vi "createPubDataEvents.vi"(8 "error in (no error)":errorcluster, 11 "PubSubDataEvent in":refnum<class "PubSubDataEvent.lvclass">) -> (0 "error out":errorcluster, 3 "PubSubDataEvent out":refnum<class "PubSubDataEvent.lvclass">)   [LabVIEW 2016, in "PubSubDataEvent.lvclass"]
uses:
  PubSubDataEvent.lvclass
  Typedefs/CommandValue.ctl
  ts_sallv_sedspectrometer/DataTypes/logevent_SettingVersions.ctl
  ts_sallv_sedspectrometer/DataTypes/logevent_SummaryState.ctl
  ts_sallv_sedspectrometer/DataTypes/logevent_RejectedCommand.ctl
  ts_sallv_sedspectrometer/DataTypes/logevent_LoopTimeOutOfRange.ctl
  ts_sallv_sedspectrometer/DataTypes/LoopTime_ms.ctl
  ts_sallv_sedspectrometer/DataTypes/logevent_Heartbeat.ctl
  ts_sallv_sedspectrometer/DataTypes/logevent_ErrorCode.ctl
  ts_sallv_sedspectrometer/DataTypes/logevent_DetailedState.ctl
  ts_sallv_sedspectrometer/DataTypes/Timestamp.ctl
  ts_sallv_sedspectrometer/DataTypes/logevent_MeasuredSpectrum.ctl
  ts_sallv_sedspectrometer/DataTypes/logevent_Timeout.ctl
  PubSubDataEvent.lvclass/PubSubDataEvent.ctl
  Typedefs/SEDSpectrometerTypedefs.lvlib
  ts_sallv_sedspectrometer/SALLV_sedSpectrometer.lvlib
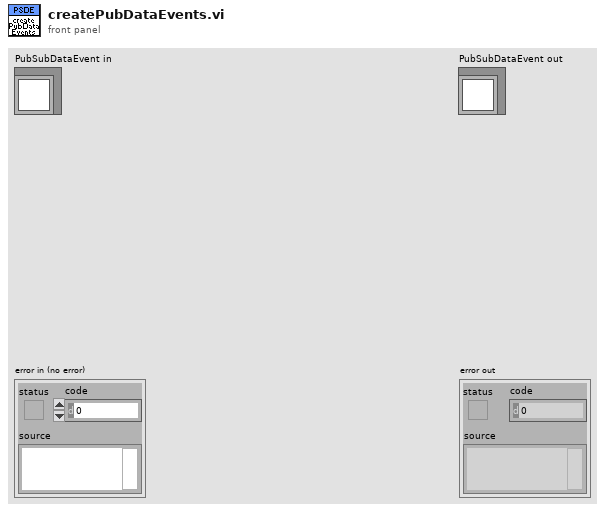
[diagram p1: front panel]
types:
  T1 = typedef "SALLV_sedSpectrometer.lvlib/logevent_Timeout.ctl" = cluster{"timeout":bool, "priority":i32}
  T2 = typedef "SALLV_sedSpectrometer.lvlib/logevent_MeasuredSpectrum.ctl" = cluster{"imageName":string, "wavelength[2048]":dbl[], "intensity[2048]":dbl[], "priority":i32}
  T3 = typedef "SALLV_sedSpectrometer.lvlib/Timestamp.ctl" = cluster{"timestamp":dbl}
  T4 = typedef "SALLV_sedSpectrometer.lvlib/logevent_DetailedState.ctl" = cluster{"detailedState":enum32{"", "DisabledState", "EnabledState", "FaultState", "OfflineState", "StandbyState"}, "priority":i32}
  T5 = typedef "SALLV_sedSpectrometer.lvlib/logevent_ErrorCode.ctl" = cluster{"errorCode":i32, "priority":i32}
  T6 = typedef "SALLV_sedSpectrometer.lvlib/logevent_Heartbeat.ctl" = cluster{"heartbeat":bool, "priority":i32}
  T7 = typedef "SALLV_sedSpectrometer.lvlib/LoopTime_ms.ctl" = cluster{"loopTime_ms":dbl}
  T8 = typedef "SALLV_sedSpectrometer.lvlib/logevent_LoopTimeOutOfRange.ctl" = cluster{"loopTimeOutOfRange":bool, "priority":i32}
  T9 = typedef "SALLV_sedSpectrometer.lvlib/logevent_RejectedCommand.ctl" = cluster{"commandValue":u16, "detailedState":u16, "timestamp":dbl, "priority":i32}
  T10 = typedef "SALLV_sedSpectrometer.lvlib/logevent_SummaryState.ctl" = cluster{"summaryState":enum32{"", "DisabledState", "EnabledState", "FaultState", "OfflineState", "StandbyState"}, "priority":i32}
  T11 = typedef "SALLV_sedSpectrometer.lvlib/logevent_SettingVersions.ctl" = cluster{"recommendedSettingsVersion":string, "recommendedSettingsLabels":string, "priority":i32}
  T12 = cluster{"appliedSettingsMatchStart":bool, "Timestamp":dbl}
  T13 = typedef "SEDSpectrometerTypedefs.lvlib/CommandValue.ctl" = enum16{"disable", "enable", "exit", "GoToStandby", "OnHeartbeat", "OnIncomingMessagingError", "OnInterrupt", "start", "captureSpectImage", "setSpectTempSetpoint", "stopImageCapture"}
  T14 = cluster{"error":i32, "result":string, "ack":i32, "cmdSeqNum":i32, "CommandValue":T13}
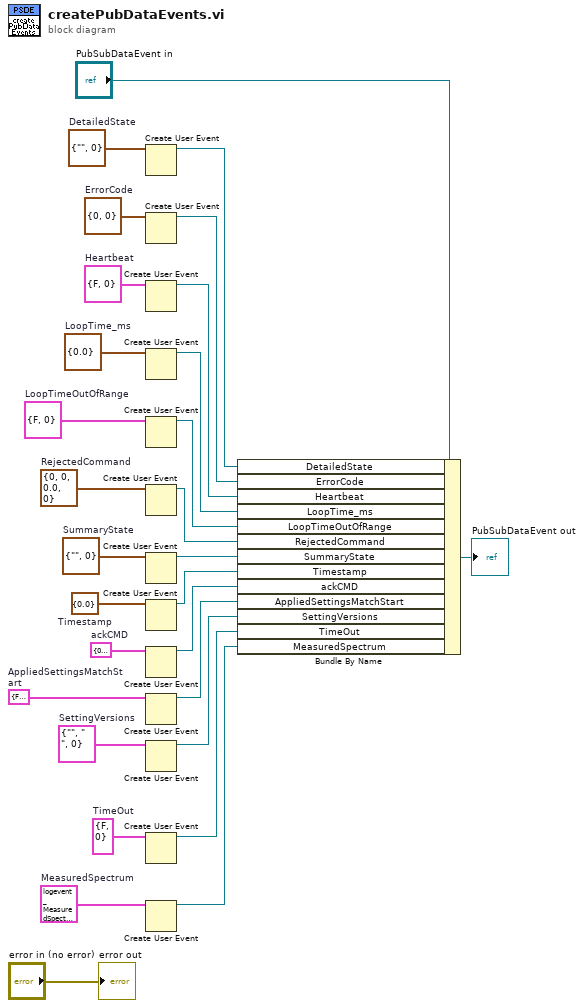
[diagram p0: block diagram]
diagram:
  w1 = T1 {"timeout"=FALSE, "priority"=0}  # TimeOut
  w2 = T2 {"imageName"="", "wavelength[2048]"=array[2048 elements], "intensity[2048]"=array[2048 elements], "priority"=0}  # MeasuredSpectrum
  w6 = T3 {"timestamp"=0.0}  # Timestamp
  w7 = T4 {"detailedState"=enum."", "priority"=0}  # DetailedState
  w8 = T5 {"errorCode"=0, "priority"=0}  # ErrorCode
  w9 = T6 {"heartbeat"=FALSE, "priority"=0}  # Heartbeat
  w11 = T7 {"loopTime_ms"=0.0}  # LoopTime_ms
  w10 = T8 {"loopTimeOutOfRange"=FALSE, "priority"=0}  # LoopTimeOutOfRange
  w13 = T9 {"commandValue"=0, "detailedState"=0, "timestamp"=0.0, "priority"=0}  # RejectedCommand
  w15 = T10 {"summaryState"=enum."", "priority"=0}  # SummaryState
  w16 = T11 {"recommendedSettingsVersion"="", "recommendedSettingsLabels"="                                                                                                                                                                                                                                                                ", "priority"=0}  # SettingVersions
  w18 = T12 {"appliedSettingsMatchStart"=FALSE, "Timestamp"=0.0}  # AppliedSettingsMatchStart
  w20 = T14 {"error"=0, "result"="", "ack"=0, "cmdSeqNum"=0, "CommandValue"=enum."disable"}  # ackCMD
  n1 = Create User Event(user event datatype=w7) -> (user event=w26:refnum<user-event>)  [unwired: 1 in, 1 out]
  n2 = Create User Event(user event datatype=w8) -> (user event=w25:refnum<user-event>)  [unwired: 1 in, 1 out]
  n3 = Create User Event(user event datatype=w9) -> (user event=w24:refnum<user-event>)  [unwired: 1 in, 1 out]
  n4 = Create User Event(user event datatype=w11) -> (user event=w23:refnum<user-event>)  [unwired: 1 in, 1 out]
  n5 = Create User Event(user event datatype=w10) -> (user event=w22:refnum<user-event>)  [unwired: 1 in, 1 out]
  n6 = Create User Event(user event datatype=w13) -> (user event=w12:refnum<user-event>)  [unwired: 1 in, 1 out]
  n7 = Create User Event(user event datatype=w15) -> (user event=w14:refnum<user-event>)  [unwired: 1 in, 1 out]
  n8 = Create User Event(user event datatype=w6) -> (user event=w21:refnum<user-event>)  [unwired: 1 in, 1 out]
  n9 = Create User Event(user event datatype=w20) -> (user event=w19:refnum<user-event>)  [unwired: 1 in, 1 out]
  n10 = Create User Event(user event datatype=w18) -> (user event=w17:refnum<user-event>)  [unwired: 1 in, 1 out]
  n11 = Create User Event(user event datatype=w16) -> (user event=w5:refnum<user-event>)  [unwired: 1 in, 1 out]
  n12 = Create User Event(user event datatype=w1) -> (user event=w4:refnum<user-event>)  [unwired: 1 in, 1 out]
  n13 = Create User Event(user event datatype=w2) -> (user event=w3:refnum<user-event>)  [unwired: 1 in, 1 out]
  n14 = Bundle By Name(cluster="PubSubDataEvent in", "DetailedState"=w26, "ErrorCode"=w25, "Heartbeat"=w24, "LoopTime_ms"=w23, "LoopTimeOutOfRange"=w22, "RejectedCommand"=w12, "SummaryState"=w14, "Timestamp"=w21, "ackCMD"=w19, "AppliedSettingsMatchStart"=w17, "SettingVersions"=w5, "TimeOut"=w4, "MeasuredSpectrum"=w3) -> (→"PubSubDataEvent out":refnum<class "PubSubDataEvent.lvclass">)
  "error out" <- "error in (no error)"
